vi "Back_End_Chiller_PID.vi"(0 "Setpoint":dbl=15.0 format="%.2f", 1 "Current Time":dbl, 2 "Previous Control Sum":dbl format="%.2f", 3 "Present Value":dbl=15.0 format="%.2f") -> (5 "Dem Output":dbl format="%.2f")   [LabVIEW 2020]
uses:
  <vilib>/Analysis/NI_AALPro.lvlib
panel:
  out "Derivative":dbl(graph)
  out "Integral":dbl(graph)
  out "Proportional":dbl(graph)
  out "Error":dbl(graph)
  in  "O/P deadband":dbl=1.0 format="%.2f"
  in  "Kp Deadband":dbl format="%.2f"
  in  "Derivative History":i32=100
  out "deadbanded error":dbl format="%.2f"
  in  "P":bool=TRUE
  in  "D":bool=TRUE
  in  "I":bool=TRUE
  in  "Manual Demand":dbl min=0.0 max=100.0 format="%.2f"
  in  "Manual Override":bool
  out "Control Sum":dbl format="%.2f"
  out "error differential":dbl format="%.5f"
  out "error integral":dbl format="%.2f"
  in  "Kd":dbl format="%.2f"
  in  "Ki":dbl=0.1 format="%.3f"
  in  "Kp":dbl=5.0 format="%.2f"
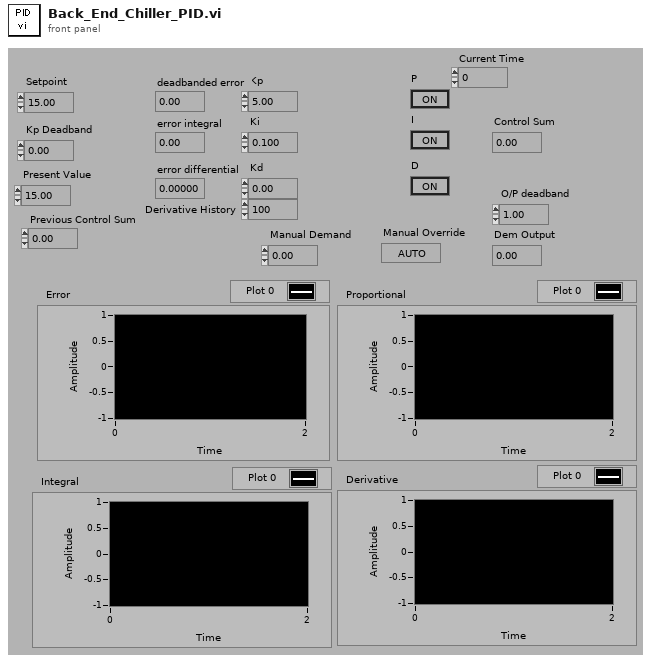
[diagram p1: front panel]
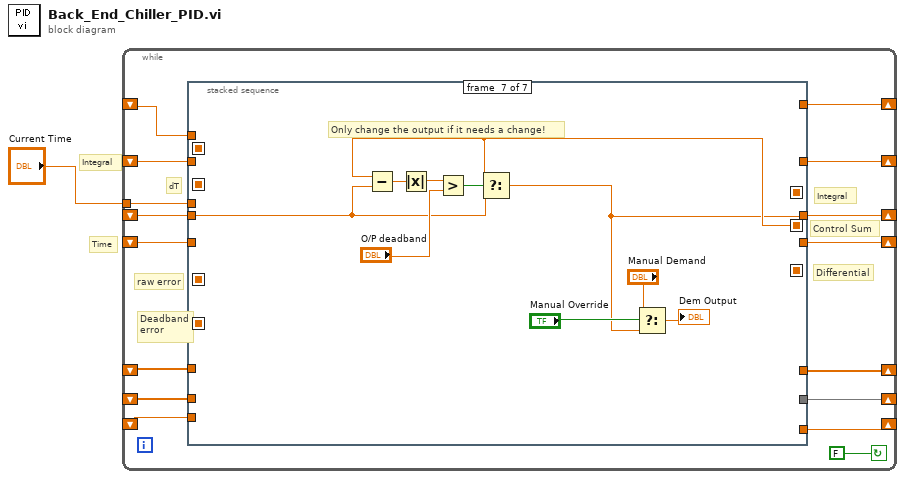
[diagram p0: block diagram]
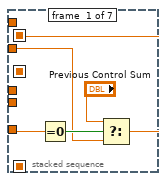
[diagram p2: hidden frame]
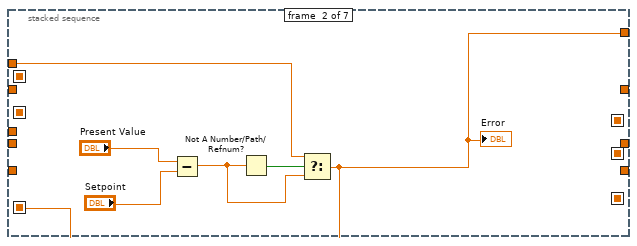
[diagram p3: hidden frame]
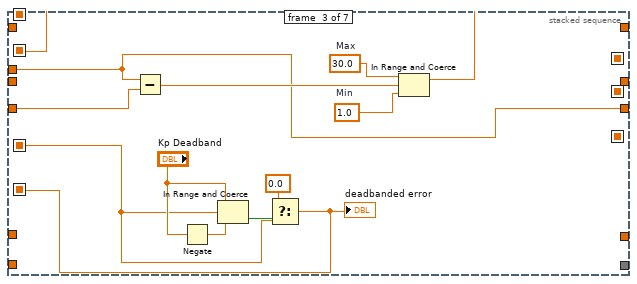
[diagram p4: hidden frame]
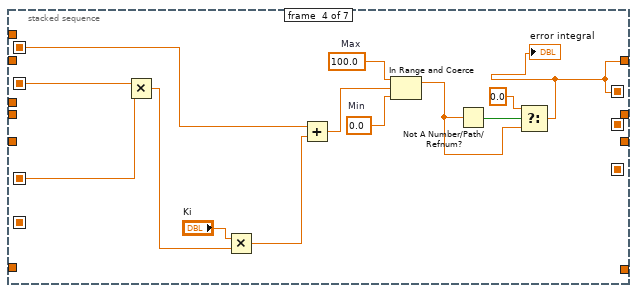
[diagram p5: hidden frame]
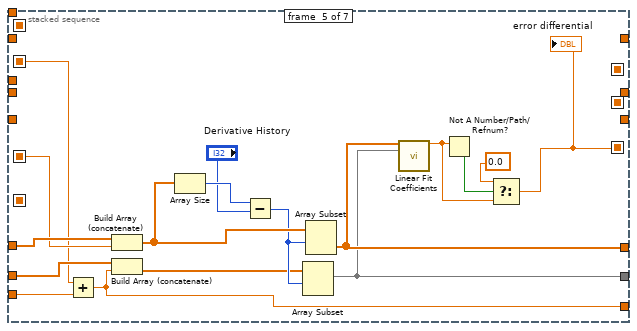
[diagram p6: hidden frame]
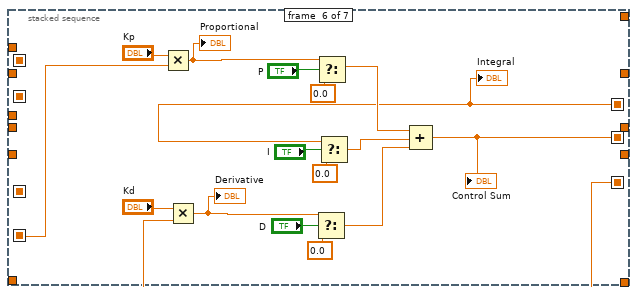
[diagram p7: hidden frame]
diagram:
  # "Integral"
  # "Time"
  n1 = while {
    shift-left: _ -> [w4]
    shift-right: [w3] -> _
    shift-left: _ -> [w6]
    shift-right: [w5] -> _
    shift-left: _ -> [w8]
    shift-right: [w7] -> _
    tunnel: "Current Time" -> [w13]
    shift-left: _ -> [w10]
    shift-right: [w9] -> _
    shift-left: _ -> [w12]
    shift-right: [w11] -> _
    shift-left: _ -> [w14]
    shift-right: [w15] -> _
    shift-left: _ -> [w17]
    shift-right: [w16] -> _
    stop <- FALSE continue-if-true
    # "Control Sum"
    # "raw error"
    # "Differential"
    # "Integral"
    # "Deadband\nerror"
    # "dT"
    n2 = stacked-sequence {
      seq-local: [_ _ w29 _ _ _ _] -> [_ _ _ w53 w56 _ _]
      seq-local: [_ _ w38 _ _ _ _] -> [_ _ _ _ _ w75 _]
      seq-local: [_ _ _ _ w61 _ _] -> [_ _ _ _ _ w74 _]
      seq-local: [_ _ _ w46 _ _ _] -> [_ _ _ _ _ w73 _]
      seq-local: [_ w23 _ _ _ _ _] -> [_ _ w30 w50 w62 _ _]
      seq-local: [_ _ _ _ _ w78 _] -> [_ _ _ _ _ _ w91]
      seq-local: [w18 _ _ _ _ _ _] -> [_ _ _ w43 _ _ _]
      tunnel: w17 -> [w22 _ w35 _ _ _ _]
      tunnel: [_ _ w33 _ _ _ _] -> w16
      tunnel: [_ _ _ w46 _ _ _] -> w15
      tunnel: w14 -> [w19 _ _ _ _ _ _]
      tunnel: w13 -> [_ _ w33 _ _ _ _]
      tunnel: w12 -> [_ _ _ _ w70 _ _]
      tunnel: [_ _ _ _ w63 _ _] -> w11
      tunnel: w10 -> [_ _ _ _ w69 _ _]
      tunnel: [_ _ _ _ w60 _ _] -> w9
      tunnel: w8 -> [_ _ _ _ _ _ w89]
      tunnel: [_ _ _ _ _ _ w88] -> w7
      tunnel: w6 -> [_ _ _ _ w55 _ _]
      tunnel: [_ _ _ _ w54 _ _] -> w5
      tunnel: w4 -> [_ w25 _ _ _ _ _]
      tunnel: [_ w23 _ _ _ _ _] -> w3
      frame #0 {
        n3 = Equal To 0?(x=w22) -> (x = 0?=w21:bool)
        n4 = Select(t="Previous Control Sum", s=w21, f=w19) -> (s? t:f=w18:dbl)
      }
      frame #1 {
        n5 = Subtract(x="Present Value", y="Setpoint") -> (x-y=w24:dbl)
        n6 = Not A Number/Path/Refnum?(number/path/refnum=w24) -> (NaN/Path/Refnum?=w26:bool)
        n7 = Select(t=w25, s=w26, f=w24) -> (s? t:f=w23:dbl)
        "Error" <- w23
      }
      frame #2 {
        w36 = 1.0  # Min
        w37 = 30.0  # Max
        n8 = Subtract(x=w33, y=w35) -> (x-y=w34:dbl)
        n9 = Negate(x="Kp Deadband") -> (-x=w32:dbl)
        n10 = In Range and Coerce(upper limit="Kp Deadband", x=w30, lower limit=w32) -> (In Range?=w39:bool)  [unwired: 1 out]
        n11 = Select(t=0.0, s=w39, f=w30) -> (s? t:f=w38:dbl)
        "deadbanded error" <- w38
        n12 = In Range and Coerce(upper limit=w37, x=w34, lower limit=w36) -> (coerced(x)=w29:dbl)  [unwired: 1 out]
      }
      frame #3 {
        w52 = 0.0  # Min
        w41 = 100.0  # Max
        n13 = Multiply(x=w53, y=w50) -> (x*y=w44:dbl)
        n14 = Multiply(x="Ki", y=w44) -> (x*y=w42:dbl)
        n15 = Add(x=w43, y=w42) -> (x+y=w51:dbl)
        n16 = In Range and Coerce(upper limit=w41, x=w51, lower limit=w52) -> (coerced(x)=w47:dbl)  [unwired: 1 out]
        n17 = Not A Number/Path/Refnum?(number/path/refnum=w47) -> (NaN/Path/Refnum?=w48:bool)
        n18 = Select(t=0.0, s=w48, f=w47) -> (s? t:f=w46:dbl)
        "error integral" <- w46
      }
      frame #4 {
        n19 = Add(x=w56, y=w55) -> (x+y=w54:dbl)
        n20 = Build Array (concatenate)(w70, w62) -> (w66:dbl[])
        n21 = Build Array (concatenate)(w69, w54) -> (w64:dbl[])
        n22 = Array Size(array=w66) -> (size(s)=w68:i32)
        n23 = Subtract(x=w68, y="Derivative History") -> (x-y=w65:i32)
        n24 = Array Subset(array=w64, index=w65) -> (w60:dbl[])  [unwired: 1 in]
        n25 = Array Subset(array=w66, index=w65) -> (w63:dbl[])  [unwired: 1 in]
        n26 = call <vilib>:"Linear Fit Coefficients.vi"("Y"=w63, "X"=w60) -> ("slope"=w57:dbl)  [unwired: 3 in, 10 out]
        n27 = Not A Number/Path/Refnum?(number/path/refnum=w57) -> (NaN/Path/Refnum?=w59:bool)
        n28 = Select(t=0.0 ("f"), s=w59, f=w57) -> (s? t:f=w61:dbl)
        "error differential" <- w61
      }
      frame #5 {
        n29 = Multiply(x="Kp", y=w75) -> (x*y=w71:dbl)
        "Proportional" <- w71
        n30 = Multiply(x="Kd", y=w74) -> (x*y=w72:dbl)
        "Derivative" <- w72
        n31 = Select(t=w72, s="D", f=0.0) -> (s? t:f=w80:dbl)
        n32 = Select(t=w71, s="P", f=0.0) -> (s? t:f=w86:dbl)
        n33 = Select(t=w73, s="I", f=0.0) -> (s? t:f=w79:dbl)
        n34 = Compound Arithmetic op=ADD(w86, w79, w80) -> (w78:dbl)
        "Control Sum" <- w78
        "Integral" <- w73
      }
      frame #6 {
        # "Only change the output if it needs a change!"
        n35 = Subtract(x=w91, y=w89) -> (x-y=w94:dbl)
        n36 = Absolute Value(x=w94) -> (abs(x)=w93:dbl)
        n37 = Greater?(x=w93, y="O/P deadband") -> (0:w92:bool)
        n38 = Select(t=w91, s=w92, f=w89) -> (s? t:f=w88:dbl)
        n39 = Select(t="Manual Demand", s="Manual Override", f=w88) -> (s? t:f=→"Dem Output":dbl)
      }
    }
  }
